vi "Register Datum When Mouse Down.vi"(8 "error in (no error)":errorcluster, 10 "Position":T1, 11 "UI Controller in":refnum<class "UI Controller.lvclass">) -> (0 "error out":errorcluster, 3 "UI Controller out":refnum<class "UI Controller.lvclass">)   [LabVIEW 2020, in "UI Controller.lvlib" / "UI Controller.lvclass"]
uses:
  UI Controller.lvclass
  <vilib>/Utility/miscctls.llb/LVPoint32TypeDef.ctl
  UI Controller.lvclass/UI Controller.ctl
  Factories/UI Factory/UI Factory.lvclass
panel:
  # "NOTICE -- YOU MUST LEAVE THIS NOTICE IN PLACE.\n\nCopyright (c) 2017, LIANG LIU Shawn.Liu.cn@gmail.com\nAll rights reserved.\n\nRedistribution and use in source and binary forms, with or without modification, are permitted provided that the following conditions are met:\n-Redistributions of source code must retain the above copyright notice, this list of conditions and the following disclaimer.\n-Redistributions in binary form must reproduce the above copyright notice, this list of conditions and the following disclaimer in the documentation and/or other materials provided with the distribution.\n-Neither the name of the eLp nor the names of its contributors may be used to endorse or promote products derived from this software without specific prior written permission.\n\nTHIS SOFTWARE IS PROVIDED BY THE COPYRIGHT HOLDERS AND CONTRIBUTORS \"AS IS\" AND ANY EXPRESS OR IMPLIED WARRANTIES, INCLUDING, BUT NOT LIMITED TO, THE IMPLIED WARRANTIES OF MERCHANTABILITY AND FITNESS FOR A PARTICULAR PURPOSE ARE DISCLAIMED. IN NO EVENT SHALL THE COPYRIGHT HOLDER OR CONTRIBUTORS BE LIABLE FOR ANY DIRECT, INDIRECT, INCIDENTAL, SPECIAL, EXEMPLARY, OR CONSEQUENTIAL DAMAGES (INCLUDING, BUT NOT LIMITED TO, PROCUREMENT OF SUBSTITUTE GOODS OR SERVICES; LOSS OF USE, DATA, OR PROFITS; OR BUSINESS INTERRUPTION) HOWEVER CAUSED AND ON ANY THEORY OF LIABILITY, WHETHER IN CONTRACT, STRICT LIABILITY, OR TORT (INCLUDING NEGLIGENCE OR OTHERWISE) ARISING IN ANY WAY OUT OF THE USE OF THIS SOFTWARE, EVEN IF ADVISED OF THE POSSIBILITY OF SUCH DAMAGE."
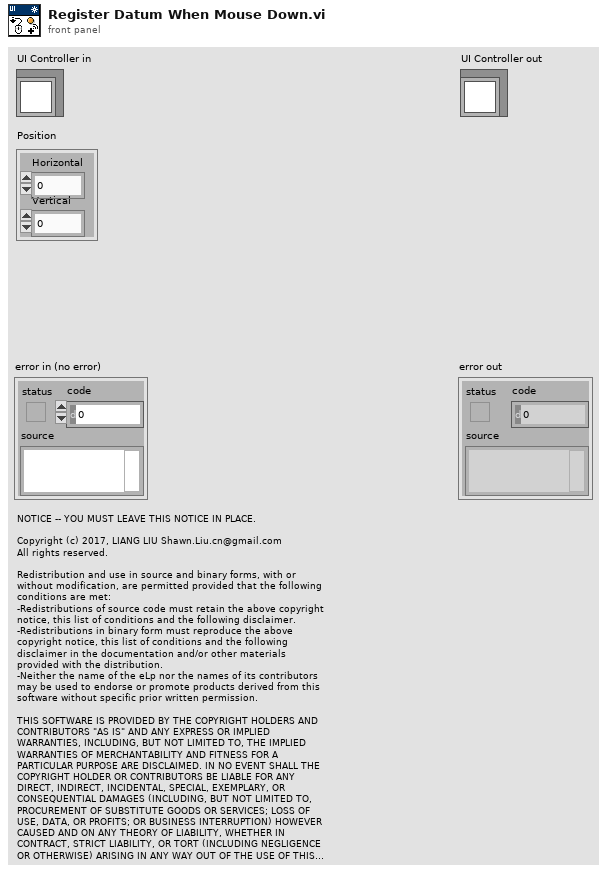
[diagram p1: front panel]
types:
  T1 = typedef "LVPoint32TypeDef.ctl" = cluster{"Horizontal":i32, "Vertical":i32}
  T2 = cluster{"left":i16, "top":i16, "right":i16, "bottom":i16}
  T3 = cluster{"Left":i16, "Top":i16, "Right":i16, "Bottom":i16}
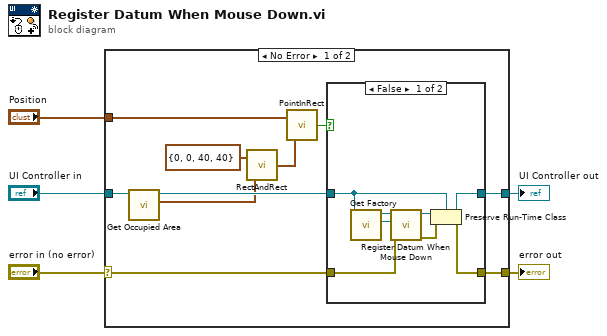
[diagram p0: block diagram]
diagram:
  n1 = case shown="No Error" "error in (no error)" {
    selector: "error in (no error)" -> [w12 w27]
    tunnel: [w15 w26] -> w5
    tunnel: [w14 w27] -> w4
    tunnel: "UI Controller in" -> [w13 w26]
    tunnel: "Position" -> [w11 _]
    frame No Error {
      n2 = call "Get Occupied Area.vi"("UI Controller in"=w13) -> ("Occupied Area"=w8:T3, "UI Controller out"=w9:refnum<class "UI Controller.lvclass">)  [unwired: 9 in]
      n3 = call <vilib>:"RectAndRect.vi"("rect b"=w8, "rect a"=T2 {"left"=0, "top"=0, "right"=40, "bottom"=40}) -> ("union rect"=w6:T2)
      n4 = call <vilib>:"PointInRect.vi"("rect"=w6, "point"=w11) -> ("pt in rect"=w10:bool)
      n5 = case shown="False" w10 {
        tunnel: w9 -> [w20 w25]
        tunnel: [w18 w25] -> w15
        tunnel: [w17 w24] -> w14
        tunnel: w12 -> [w16 w24]
        frame False {
          n6 = call "Get Factory.vi"("UI Controller in"=w20) -> ("Factory"=w21:refnum<class "UI Factory.lvclass">, "UI Controller out"=w23:refnum<class "UI Controller.lvclass">)  [unwired: 9 in]
          n7 = call-dynamic "Register Datum When Mouse Down.vi"("error in (no error)"=w16, "UI Factory in"=w21, "UI Controller in"=w23) -> ("error out"=w19:errorcluster, "UI Controller out"=w22:refnum<class "UI Controller.lvclass">)  [unwired: 7 in]
          n8 = Preserve Run-Time Class(object in=w22, error in=w19, 2:w20) -> (object out=w18:refnum<class "UI Controller.lvclass">, error out=w17:errorcluster)
        }
        frame True {
        }
      }
    }
    frame Error {
    }
  }
  "error out" <- w4
  "UI Controller out" <- w5
